vi "Cleanup.vi"(8 "error in (no error)":errorcluster, 11 "Service Container in":refnum<class "Service Container.lvclass">) -> (0 "error out":errorcluster)   [LabVIEW 2020]
uses:
  Service Container.lvclass
  C:/dev/lv20CE/lv-vecto/Vecto/Service Container/Service Container.lvclass
  C:/Program Files (x86)/National Instruments/LabVIEW 2020/vi.lib/IlluminatedG/IG HTTP Server/HTTP Server/Service/Service.lvclass
  Service/Service.lvclass
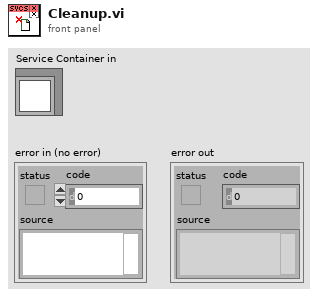
[diagram p1: front panel]
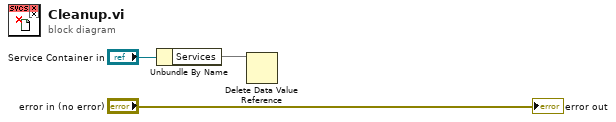
[diagram p0: block diagram]
diagram:
  n1 = Unbundle By Name("Service Container in") -> ("Services"=w1)
  n2 = Delete Data Value Reference(data value reference=w1) -> ()  [unwired: 1 in, 2 out]
  "error out" <- "error in (no error)"
